vi "S2DS_ConfigWriteWC (SubVI).vi"(6 "error in (no error)":errorcluster, 8 "WC info list":T2, 9 "Refnum in":T1) -> (0 "error out":errorcluster, 3 "Refnum out":T1)   [LabVIEW 2025]
uses:
  <vilib>/Utility/config.llb/Config Data RefNum.ctl
  TYPE DEFS/S2DS_WC info.ctl
  TYPE DEFS/S2DS_Single WC info.ctl
  <vilib>/Utility/config.llb/Write Key (U32).vi
  <vilib>/Utility/config.llb/Write Key (String).vi
  <vilib>/Utility/config.llb/Write Key (Double).vi
  <vilib>/Utility/config.llb/NI_LVConfig.lvlib
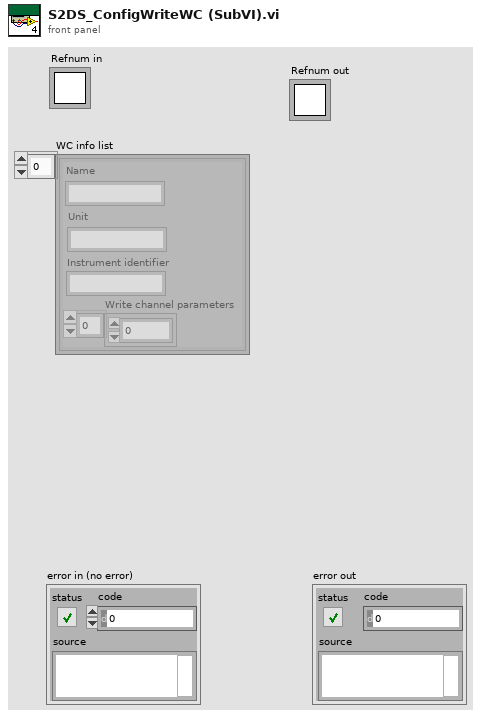
[diagram p1: front panel]
types:
  T1 = typedef "NI_LVConfig.lvlib/Config Data RefNum.ctl" = refnum<k1>
  T2 = typedef "S2DS_WC info.ctl" = T3[]
  T3 = typedef "S2DS_Single WC info.ctl" = cluster{"Instrument identifier":string, "Write channel parameters":dbl[], "Name":string, "Unit":string}
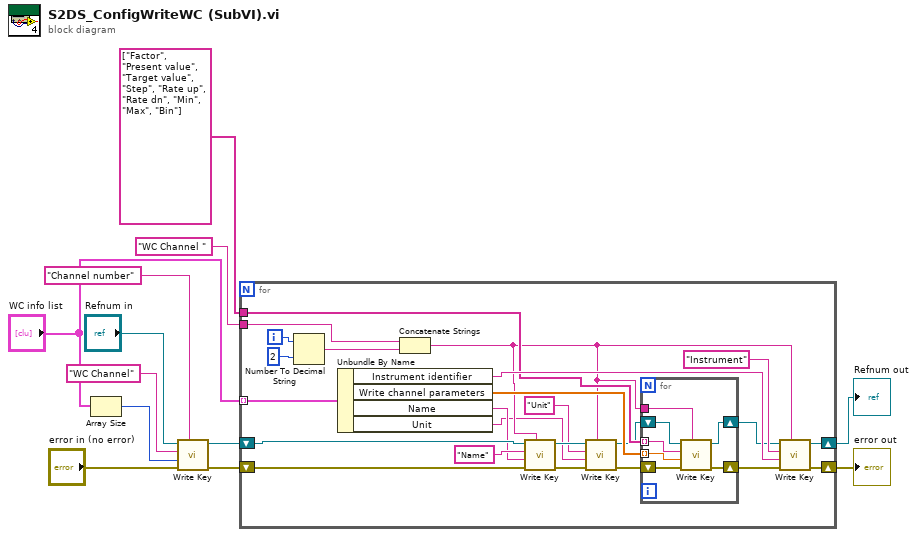
[diagram p0: block diagram]
diagram:
  n1 = Array Size(array="WC info list") -> (size(s)=w5:i32)
  n2 = call-poly <vilib>:"Write Key.vi"("section"="Channel number", "error in (no error)"="error in (no error)", "value"=w5, "key"="WC Channel", "refnum"="Refnum in") -> ("error out"=w1:errorcluster, "refnum out"=w2:T1)  [unwired: 4 in, 1 out]
  n3 = for {
    tunnel: "WC Channel " -> [w36]
    shift-right: [w16] -> w11
    shift-left: w2 -> [w28]
    tunnel: "WC info list" -> [w33] mode=indexing
    shift-right: [w17] -> w12
    shift-left: w1 -> [w27]
    tunnel: string[] ["Factor", "Present value", "Target value", "Step", "Rate up", "Rate dn", "Min", "Max", "Bin"] -> [w29]
    i -> [w15]
    n4 = Number To Decimal String(number=w15, width (-)=i16 2) -> (decimal integer string=w34:string)
    n5 = Unbundle By Name(w33) -> ("Instrument identifier"=w31:string, "Write channel parameters"=w30:dbl[], "Name"=w14:string, "Unit"=w13:string)
    n6 = Concatenate Strings(w36, w34) -> (w22:string)
    n7 = call-poly <vilib>:"Write Key.vi"("section"=w22, "error in (no error)"=w27, "value"=w14, "key"="Name", "refnum"=w28) -> ("error out"=w24:errorcluster, "refnum out"=w25:T1)  [unwired: 4 in, 1 out]
    n8 = call-poly <vilib>:"Write Key.vi"("section"=w22, "error in (no error)"=w24, "value"=w13, "key"="Unit", "refnum"=w25) -> ("error out"=w20:errorcluster, "refnum out"=w21:T1)  [unwired: 4 in, 1 out]
    n9 = for {
      tunnel: w30 -> [w38] mode=indexing
      tunnel: w29 -> [w39] mode=indexing
      shift-right: [w42] -> w19
      shift-left: w21 -> [w43]
      shift-right: [w40] -> w18
      shift-left: w20 -> [w41]
      tunnel: w22 -> [w37]
      n10 = call-poly <vilib>:"Write Key.vi"("section"=w37, "error in (no error)"=w41, "value"=w38, "key"=w39, "refnum"=w43) -> ("error out"=w40:errorcluster, "refnum out"=w42:T1)  [unwired: 4 in, 1 out]
    }
    n11 = call-poly <vilib>:"Write Key.vi"("section"=w22, "error in (no error)"=w18, "value"=w31, "key"="Instrument", "refnum"=w19) -> ("error out"=w17:errorcluster, "refnum out"=w16:T1)  [unwired: 4 in, 1 out]
  }
  "error out" <- w12
  "Refnum out" <- w11
